vi "AlignPhases.vi"(8 "error in (no error)":errorcluster, 11 "C37.118 PMU in":refnum<class "C37.118 PMU.lvclass">) -> (0 "error out":errorcluster, 3 "C37.118 PMU out":refnum<class "C37.118 PMU.lvclass">, 4 "PhaseArray":T1[](array[typedef]))   [LabVIEW 2014, in "SensorPlugins.lvlib" / "C37.118 PMU.lvclass"]
uses:
  C37.118 PMU.lvclass
  PmuBaseClass/Typedef/ePhases.ctl
  C37.118 PMU.lvclass/C37.118 PMU.ctl
  PmuBaseClass/PmuBase.lvclass/PmuBase.ctl
  PmuBaseClass/Accessors/Write PhaseArray.vi
  Accessors/Read PMUConfigData.vi
  PmuBaseClass/Accessors/Read PhaseArray.vi
  PmuBaseClass/PmuBase.lvclass
panel:
  in  "BtnDone":bool
  in  "Phases":T1[](array[typedef])=[enum."VA", enum."VB", enum."VC", enum."V+", enum."IA", enum."IB", enum."IC", enum."I+"]
  out "Channel Names":string[](array[string])
  # "Select the PMU Phases\nto match the channel \nnames"
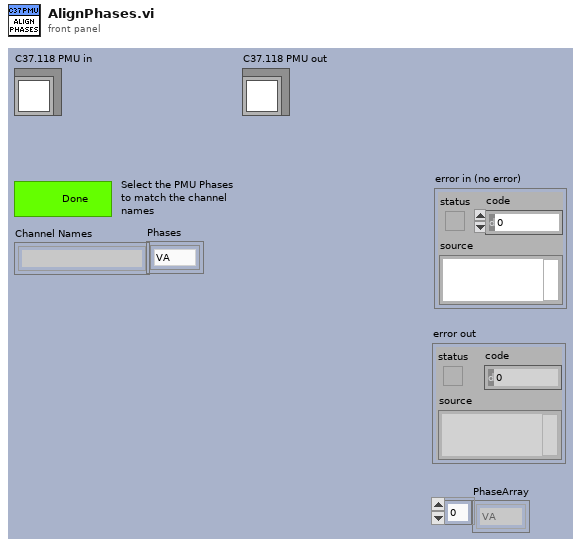
[diagram p1: front panel]
types:
  T1 = typedef "SensorPlugins.lvlib/PmuBase.lvclass/ePhases.ctl" = enum16{"VA", "VB", "VC", "V+", "IA", "IB", "IC", "I+", "none"}
  T2 = enum32{"Invalid", "Standard", "Closed", "Hidden", "Minimized", "Maximized"}
  T3 = enum32{"Invalid", "Default", "Floating", "Floating/Auto-Hide", "Modal"}
  T4 = typedef "SensorPlugins.lvlib/C37.118 PMU.lvclass/PMUConfigData.ctl" = cluster{"TimeBase":u32, "NUM_PMU":u16, "Station Name":string, "IDCODE":u16, "PHRNMR":u16, "ANNMR":u16, "DIGNMR":u16, "FORMAT BITS":T5, "Valid Inputs":u16[], "DigitalStatusMask":u16[], "24bit_PHUNIT":i32[], "24bit_ANUNIT":u32[], "Analog Amplitude Setting":u32[], "Unit (Vor I)":u8[], "ChannelNames":string, "Fs":i16, "SOC ":u32, "FRACSEC":u32, "F0":sgl, "CFGCNT":u16}
  T5 = typedef "SensorPlugins.lvlib/C37.118 PMU.lvclass/FormatBits.ctl" = cluster{"Rect/Polar":bool, "Phasor Int/Float":bool, "Analog Int/Float":bool, "F/ROCOF Int/Float":bool}
  T6 = typedef "LVRectTypeDef.ctl" = cluster{"Left":i16, "Top":i16, "Right":i16, "Bottom":i16}
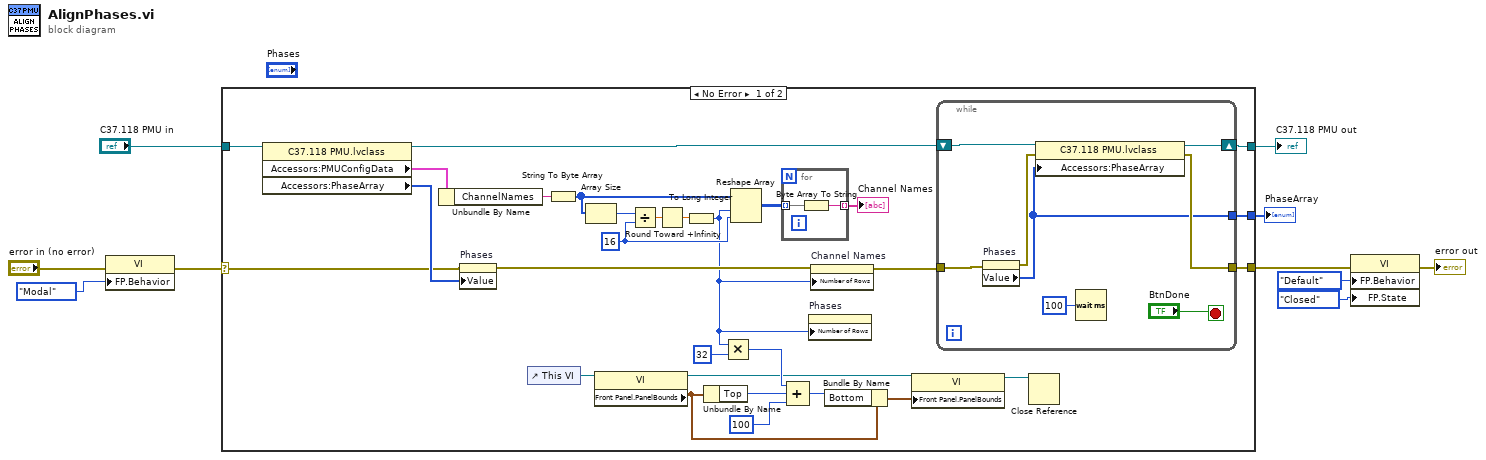
[diagram p0: block diagram]
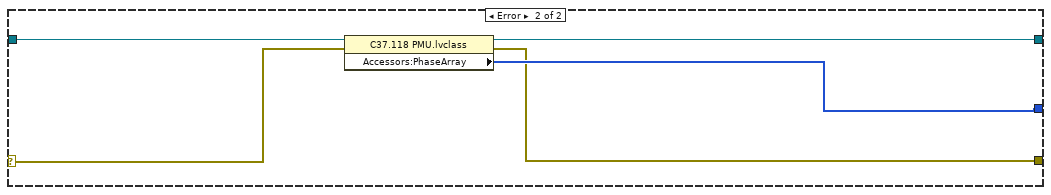
[diagram p2: hidden frame]
diagram:
  n1 = property class="VI"(error in="error in (no error)", "FP.Behavior"=T3."Modal" ("Front Panel Window:Behavior")) -> (error out=w6:errorcluster)  [unwired: 1 in, 1 out]
  n2 = case shown="No Error" w6 {
    selector: w6 -> [w25 w51]
    tunnel: [w27 w50] -> w4
    tunnel: [w28 w53] -> w9
    tunnel: "C37.118 PMU in" -> [w39 w54]
    tunnel: [w24 w52] -> w8
    frame No Error {
      w30 = 16 ("dimension size")
      n3 = property class="C37.118 PMU.lvclass"(reference=w39) -> (reference out=w29:refnum<class "C37.118 PMU.lvclass">, "Accessors:PMUConfigData"=w38:T4, "Accessors:PhaseArray"=w26:T1[])  [unwired: 1 in, 1 out]
      n4 = Unbundle By Name(w38) -> ("ChannelNames"=w37:string)
      n5 = property on="Phases" class="Arr (strict)"(error in=w25, "Value"=w26) -> (error out=w23:errorcluster)  [unwired: 1 in, 1 out]
      n6 = control-ref of="This VI"() -> (w21:refnum<vi>)
      n7 = String To Byte Array(string=w37) -> (unsigned byte array=w36:u8[])
      n8 = Array Size(array=w36) -> (size(s)=w35:i32)
      n9 = property class="VI"(reference=w21) -> (reference out=w17:refnum<vi>, "Front Panel.PanelBounds"=w16:T6)  [unwired: 1 in, 1 out]
      n10 = Divide(x=w35, y=w30) -> (x/y=w34:dbl)
      n11 = Round Toward +Infinity(x=w34) -> (ceil(x): smallest int >= x=w33:dbl)
      n12 = To Long Integer(number=w33) -> (32bit integer=w11:i32)
      n13 = Unbundle By Name(w16) -> ("Top"=w20:i16)
      n14 = Multiply(x=w11, y=32) -> (x*y=w18:i32)
      n15 = Reshape Array(w36, w11, w30) -> (w32:u8[][])
      n16 = for {
        tunnel: w32 -> [w49] mode=indexing
        tunnel: [w48] -> w31 mode=indexing
        n17 = Byte Array To String(unsigned byte array=w49) -> (string=w48:string)
      }
      "Channel Names" <- w31
      n18 = Compound Arithmetic op=ADD(w18, w20, i16 100 ("value")) -> (w15:i32)
      n19 = property on="Phases" class="Arr (strict)"("Number of Rows"=w11) -> ()  [unwired: 2 in, 2 out]
      n20 = property on="Channel Names" class="Arr (strict)"(error in=w23, "Number of Rows"=w11) -> (error out=w22:errorcluster)  [unwired: 1 in, 1 out]
      n21 = Bundle By Name(cluster=w16, "Bottom"=w15) -> (w14:T6)
      n22 = property class="VI"(reference=w17, "Front Panel.PanelBounds"=w14) -> (reference out=w13:refnum<vi>)  [unwired: 1 in, 1 out]
      n23 = while {
        shift-right: [w46] -> w28
        shift-left: w29 -> [w47]
        tunnel: [w44] -> w24
        tunnel: w22 -> [w43]
        tunnel: [w45] -> w27
        stop <- "BtnDone" stop-if-true
        n24 = property on="Phases" class="Arr (strict)"(error in=w43) -> (error out=w42:errorcluster, "Value"=w44:T1[])  [unwired: 1 in, 1 out]
        n25 = property class="C37.118 PMU.lvclass"(reference=w47, error in=w42, "Accessors:PhaseArray"=w44) -> (reference out=w46:refnum<class "C37.118 PMU.lvclass">, error out=w45:errorcluster)
        n26 = Wait (ms)(milliseconds to wait=u32 100) -> ()  [unwired: 1 out]
      }
      n27 = Close Reference(reference=w13) -> ()  [unwired: 1 in, 1 out]
    }
    frame Error {
      n28 = property class="C37.118 PMU.lvclass"(reference=w54, error in=w51) -> (reference out=w53:refnum<class "C37.118 PMU.lvclass">, error out=w50:errorcluster, "Accessors:PhaseArray"=w52:T1[])
    }
  }
  "C37.118 PMU out" <- w9
  "PhaseArray" <- w8
  n29 = property class="VI"(error in=w4, "FP.Behavior"=T3."Default" ("Front Panel Window:Behavior"), "FP.State"=T2."Closed" ("Front Panel Window:State")) -> (error out=→"error out":errorcluster)  [unwired: 1 in, 1 out]
